vi "Split Console.vi"(11 "Console":string) -> (2 "Dongle":string, 3 "Spike":string)   [LabVIEW 2020]
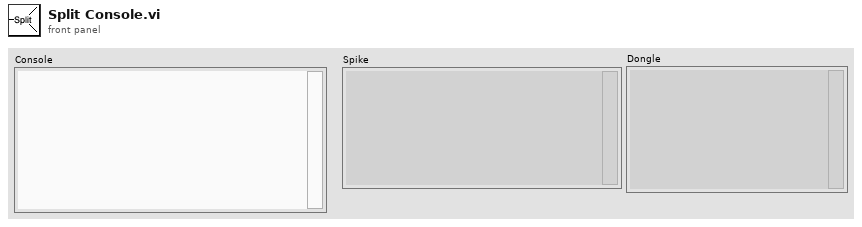
[diagram p1: front panel]
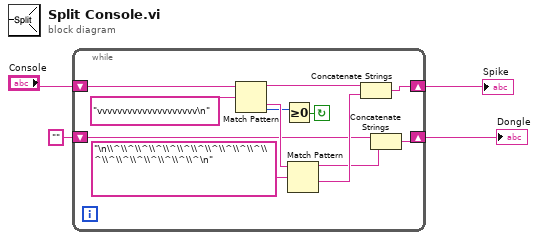
[diagram p0: block diagram]
diagram:
  n1 = while {
    shift-right: [w16] -> w4
    shift-left: "Console" -> [w12]
    shift-right: [w7] -> w3
    shift-left: "" -> [w9]
    stop <- w5 continue-if-true
    n2 = Match Pattern(string=w12, regular expression="vvvvvvvvvvvvvvvvvvvv\n") -> (before substring=w14:string, after substring=w11:string, offset past match=w6:i32)  [unwired: 1 in, 1 out]
    n3 = Greater Or Equal To 0?(x=w6) -> (x >= 0?=w5:bool)
    n4 = Match Pattern(string=w11, regular expression="\n\\^\\^\\^\\^\\^\\^\\^\\^\\^\\^\\^\\^\\^\\^\\^\\^\\^\\^\\^\n") -> (before substring=w8:string, after substring=w15:string)  [unwired: 1 in, 2 out]
    n5 = Concatenate Strings(w14, w15) -> (w16:string)
    n6 = Concatenate Strings(w9, w8) -> (w7:string)
  }
  "Spike" <- w4
  "Dongle" <- w3
